vi "Copy Encoding Errors to Built Directory.vi"(6 "Top Level/Always Included VIs":path[](array[path]), 7 "Main Destination Path":path, 9 "Target Name":string, 10 "Build Specification Name":string, 11 "Project Path":path) -> (0 "error out":errorcluster)   [LabVIEW 2020]
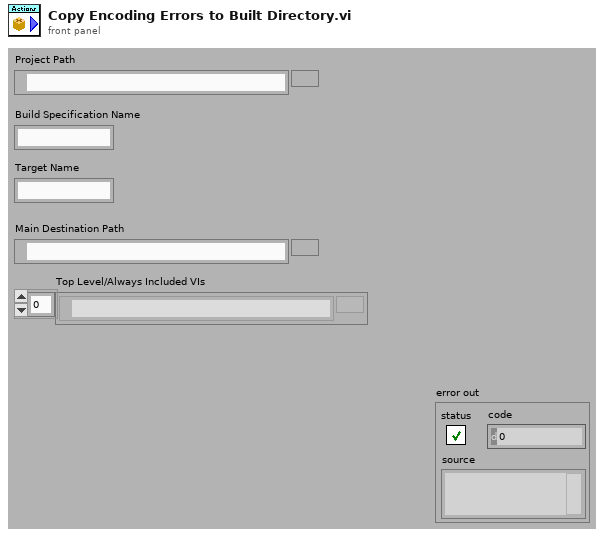
[diagram p1: front panel]
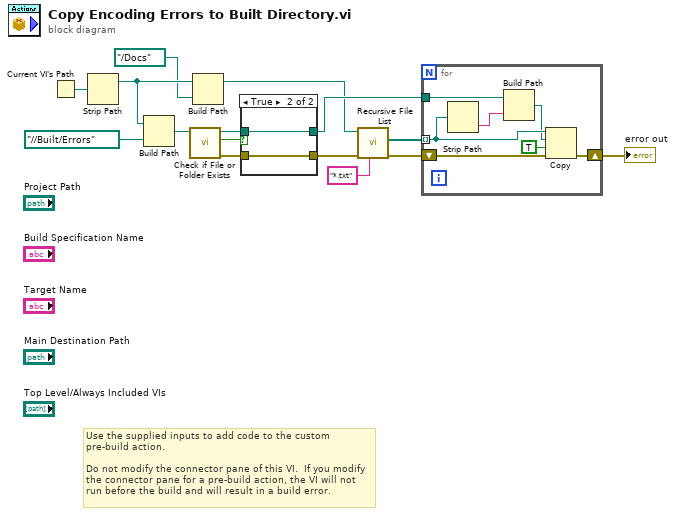
[diagram p0: block diagram]
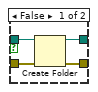
[diagram p2: hidden frame]
diagram:
  # "Use the supplied inputs to add code to the custom pre-build action.\n\nDo not modify the connector pane of this VI.  If you modify the connector pane for a pre-build action, the VI will not run before the build and will result in a build error."
  n1 = Current VI's Path() -> (path=w15:path)
  n2 = Strip Path(path=w15) -> (stripped path=w2:path)  [unwired: 1 out]
  n3 = Build Path(base path=w2, name or relative path=path "../../Built/Errors" ("stripped path")) -> (appended path=w10:path)
  n4 = call <vilib>:"Check if File or Folder Exists.vi"("path"=w10) -> ("error out"=w8:errorcluster, "file or folder exists?"=w9:bool, "dup path"=w7:path)  [unwired: 8 in]
  n5 = Build Path(base path=w2, name or relative path=path "../Docs") -> (appended path=w3:path)
  n6 = case shown="True" w9 {
    tunnel: w8 -> [w18 w21]
    tunnel: w7 -> [w19 w20]
    tunnel: [w17 w21] -> w6
    tunnel: [w16 w20] -> w5
    frame False {
      n7 = Create Folder(path (use dialog)=w19, error in=w18) -> (created path=w16:path, error out=w17:errorcluster)  [unwired: 1 in, 1 out]
    }
    frame True {
    }
  }
  n8 = call <vilib>:"Recursive File List.vi"("pattern"="*.txt", "error in (no error)"=w6, "Folder Path"=w3) -> ("error out"=w12:errorcluster, "All Files in Dir"=w13:path[])  [unwired: 4 in, 3 out]
  n9 = for {
    tunnel: w13 -> [w26] mode=indexing
    tunnel: w5 -> [w27]
    shift-right: [w22] -> w4
    shift-left: w12 -> [w28]
    n10 = Strip Path(path=w26) -> (name=w25:string)  [unwired: 1 out]
    n11 = Build Path(base path=w27, name or relative path=w25) -> (appended path=w24:path)
    n12 = Copy(8:w28, 9:TRUE ("overwrite (F)"), 10:w24, 11:w26) -> (0:w22:errorcluster)  [unwired: 1 in, 2 out]
  }
  "error out" <- w4
